vi "Send SetSyncTrigger.vi"(7 "Message Priority (Normal)":T1=enum."Normal", 8 "error in (no error)":errorcluster, 9 "SyncLevel":i32=-100 caption="Level      mV" min=-1200 max=1200 step=1, 10 "SyncEdge":i32(ring) caption="Edge" items=["falling", "rising"], 11 "Message Enqueuer":refnum<class "Message Enqueuer.lvclass">) -> (0 "error out":errorcluster, 3 "Message Enqueuer out":refnum<class "Message Enqueuer.lvclass">)   [LabVIEW 2023, in "Multiharp.lvlib" / "SetSyncTrigger Msg.lvclass"]
doc: "This VI sends the message to an actor."
uses:
  SetSyncTrigger Msg.lvclass
  <vilib>/ActorFramework/Message Enqueuer/Message Enqueuer.lvclass
  C:/Program Files/National Instruments/LabVIEW 2023/vi.lib/ActorFramework/Message/Message.lvclass
  C:/Users/PC/Documents/SinglePhotonInterferometry/Multiharp/Multiharp Messages/SetSyncTrigger Msg/SetSyncTrigger Msg.lvclass
  <vilib>/ActorFramework/Message Enqueuer/Message Priority.ctl
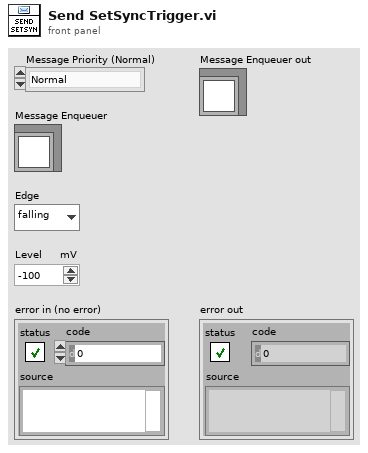
[diagram p1: front panel]
types:
  T1 = typedef "Actor Framework.lvlib/Message Enqueuer.lvclass/Message Priority.ctl" = enum16{"Low", "Normal", "High"}
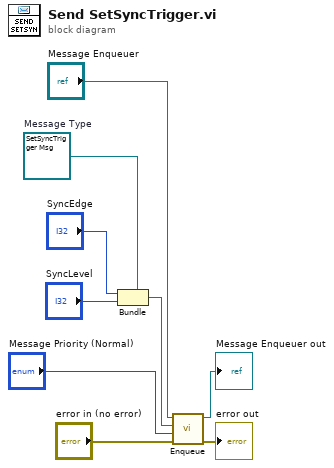
[diagram p0: block diagram]
diagram:
  w3 = refnum<class "SetSyncTrigger Msg.lvclass"> refnum  # Message Type
  n1 = Bundle(cluster=w3, "SyncEdge", "SyncLevel") -> (w4:refnum<class "SetSyncTrigger Msg.lvclass">)
  n2 = call <vilib>:"Enqueue.vi"("error in (no error)"="error in (no error)", "Message Priority (Normal)"="Message Priority (Normal)", "Message"=w4, "Message Enqueuer in"="Message Enqueuer") -> ("error out"=→"error out":errorcluster, "Message Enqueuer out"=→"Message Enqueuer out":refnum<class "Message Enqueuer.lvclass">)  [unwired: 6 in]
